vi "Update settings.vi"(8 "error in (no error)":errorcluster) -> (0 "error out":errorcluster)   [LabVIEW 2016]
uses:
  General/Controls/Queue modes.ctl
  General/Controls/State control cluster.ctl
  General/Controls/States.ctl
  Controls/Command cluster.ctl
  Controls/Command list.ctl
  Controls/Actuator fgv modes.ctl
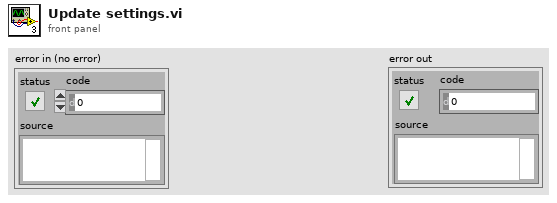
[diagram p1: front panel]
types:
  T1 = typedef "Command cluster.ctl" = cluster{"Command":T2, "data":variant}
  T2 = typedef "Command list.ctl" = enum16{"", "£nabort", "getaxisno", "£getserialno", "£nidentify", "&&£setnlimit", "&£nm", "&£snv", "&£speed", "£np", "£ncal"}
  T3 = typedef "Actuator fgv modes.ctl" = enum16{"Initalise", "COM", "Limit", "Speed", "Home", "Get"}
  T4 = typedef "State control cluster.ctl" = cluster{"State":T5, "Data":variant}
  T5 = typedef "States.ctl" = enum16{"Initialise", "Actuator connection", "Get info", "Send command", "Load method", "Run method", "Save test", "Setup", "Shutdown"}
  T6 = typedef "Queue modes.ctl" = enum16{"Initialise", "Destroy", "Get"}
  T7 = typedef "Default settings.ctl" = cluster{"COM port":refnum<visa-resource-name>, "Home pos":dbl, "Speed":dbl, "Limit stop":dbl}
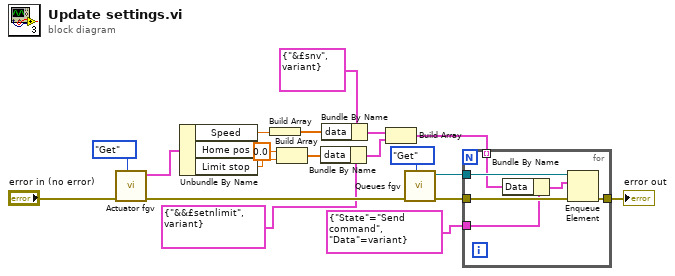
[diagram p0: block diagram]
diagram:
  n1 = call "Actuator fgv.vi"("Enum"=Actuator_fgv_modes."Get", "error in (no error)"="error in (no error)") -> ("error out"=w17:errorcluster, "Cluster out"=w19:T7)  [unwired: 8 in]
  n2 = Unbundle By Name(w19) -> ("Speed"=w14:dbl, "Limit stop"=w5:dbl)  [unwired: 1 out]
  n3 = Build Array(w14) -> (w13:dbl[])
  n4 = Build Array(0.0 ("element"), w5) -> (w4:dbl[])
  n5 = Bundle By Name(cluster=T1 {"Command"=enum."&&£setnlimit", "data"=variant} ("Cluster"), "data"=w4) -> (w3:T1)
  n6 = Bundle By Name(cluster=T1 {"Command"=enum."&£snv", "data"=variant} ("Cluster"), "data"=w13) -> (w10:T1)
  n7 = Build Array(w10, w3) -> (w9:T1[])
  n8 = call "Queues fgv.vi"("Modes"=Queue_modes."Get", "error in (no error)"=w17) -> ("error in (no error) 2"=w16:errorcluster, "Ivium"=w12:refnum<queue>)  [unwired: 6 in, 2 out]
  n9 = for {
    tunnel: w16 -> [w25]
    tunnel: w12 -> [w24]
    tunnel: T4 {"State"=enum."Send command", "Data"=variant} ("element") -> [w23]
    tunnel: w9 -> [w22] mode=indexing
    tunnel: [w20] -> w6
    n10 = Bundle By Name(cluster=w23, "Data"=w22) -> (w21:T4)
    n11 = Enqueue Element(queue=w24, element=w21, error in (no error)=w25) -> (error out=w20:errorcluster)  [unwired: 1 in, 2 out]
  }
  "error out" <- w6
